vi "CRYRead Range.vi"(1 "In s<->Hz":bool) -> (0 "Out Search_Range":string[](array[string]))   [LabVIEW 2013]
uses:
  CRYMainGlobal.vi
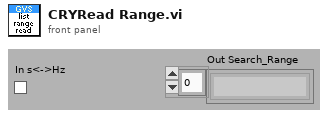
[diagram p1: front panel]
types:
  T1 = enum16{"open", "replace", "create", "open or create", "replace or create", "replace or create with confirmation"}
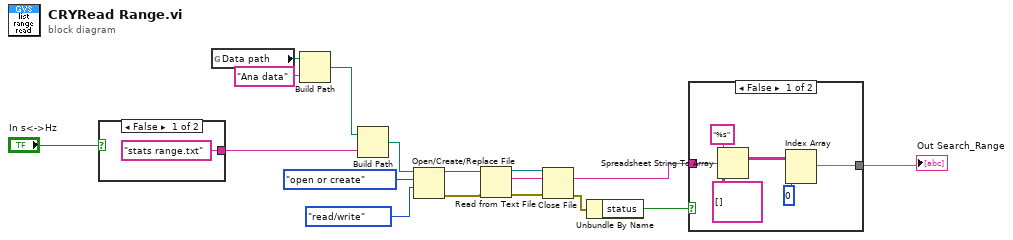
[diagram p0: block diagram]
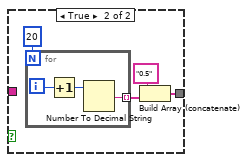
[diagram p2: hidden frame]
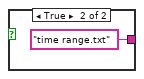
[diagram p3: hidden frame]
diagram:
  n1 = case shown="False" "In s<->Hz" {
    tunnel: ["stats range.txt" ("name or relative path") "time range.txt" ("name or relative path")] -> w10
    frame False {
    }
    frame True {
    }
  }
  n2 = global read "CRYMainGlobal.vi" "Data path"() -> (w5:path)
  n3 = Build Path(base path=w5, name or relative path="Ana data") -> (appended path=w6:path)
  n4 = Build Path(base path=w6, name or relative path=w10) -> (appended path=w9:path)
  n5 = Open/Create/Replace File(file path (use dialog)=w9, operation (0:open)=T1."open or create", access (0:read/write)=enum16{"read/write", "read-only", "write-only"}."read/write") -> (refnum out=w14:refnum<file>, error out=w15:errorcluster)  [unwired: 1 in, 3 out]
  n6 = Read from Text File(file (use dialog)=w14, error in=w15) -> (refnum out=w16:refnum<file>, text=w2:string, error out=w8:errorcluster)  [unwired: 1 in, 2 out]
  n7 = Close File(refnum=w16, error in=w8) -> (error out=w4:errorcluster)  [unwired: 1 out]
  n8 = Unbundle By Name(w4) -> ("status"=w3:bool)
  n9 = case shown="False" w3 {
    tunnel: w2 -> [w22 _]
    tunnel: [w19 w25] -> w1
    frame False {
      n10 = Spreadsheet String To Array(format string="%s", spreadsheet string=w22, array type (2D Dbl)=string[][] []) -> (array=w20:string[][])  [unwired: 1 out]
      n11 = Index Array(array=w20, index (col)=0 ("Index")) -> (element=w19:string[])  [unwired: 1 in]
    }
    frame True {
      n12 = for {
        N: 20 -> [_]
        tunnel: [w29] -> w28 mode=indexing
        i -> [w31]
        n13 = Increment(x=w31) -> (x+1=w30:i32)
        n14 = Number To Decimal String(number=w30) -> (decimal integer string=w29:string)  [unwired: 1 out]
      }
      n15 = Build Array (concatenate)("0.5", w28) -> (w25:string[])
    }
  }
  "Out Search_Range" <- w1
